vi "BRig_FPGA_stateSelection_laserEvent.vi"(0 "I_LR_reward":bool, 1 "I_LR_reward_laser":bool, 3 "I_LR_wrong":bool, 4 "I_LR_wrong_laser":bool, 6 "I_selectWrong":bool, 7 "laser_reward_nTotal":u32=100, 8 "I_selectReward":bool, 9 "laser_reward_nDelay":u32, 10 "counter":u32, 11 "laser_wrong_nTotal":u32=100, 13 "laser_wrong_nDelay":u32) -> (12 "output_counter":u32, 15 "output_I_laserEvent":bool, 17 "output_I_laserOn":bool)   [LabVIEW 2014]
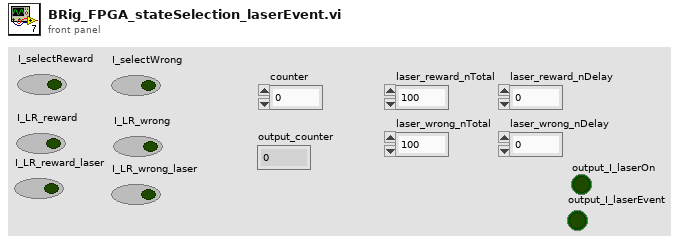
[diagram p1: front panel]
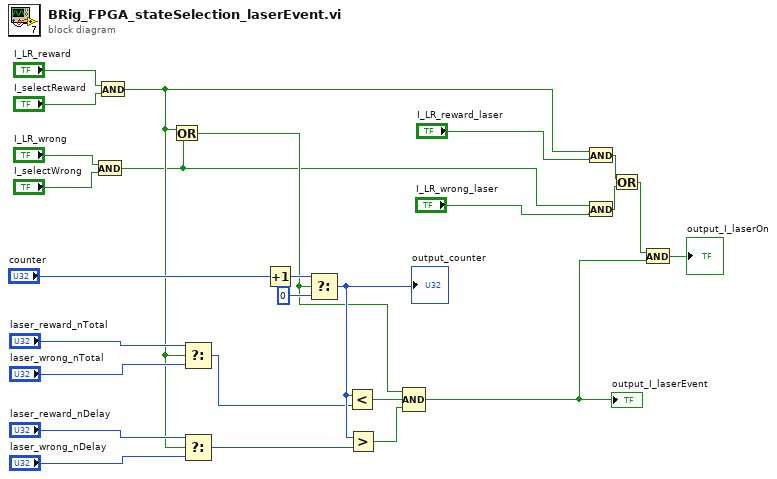
[diagram p0: block diagram]
diagram:
  n1 = And(x="I_LR_wrong", y="I_selectWrong") -> (x .and. y?=w6:bool)
  n2 = And(x="I_LR_reward", y="I_selectReward") -> (x .and. y?=w9:bool)
  n3 = Or(x=w9, y=w6) -> (x .or. y?=w10:bool)
  n4 = Select(t="laser_reward_nTotal", s=w9, f="laser_wrong_nTotal") -> (s? t:f=w13:u32)
  n5 = Select(t="laser_reward_nDelay", s=w9, f="laser_wrong_nDelay") -> (s? t:f=w18:u32)
  n6 = Increment(x="counter") -> (x+1=w22:u32)
  n7 = Select(t=w22, s=w10, f=u32 0) -> (s? t:f=w19:u32)
  "output_counter" <- w19
  n8 = Less?(x=w19, y=w13) -> (x < y?=w11:bool)
  n9 = Greater?(x=w19, y=w18) -> (0:w12:bool)
  n10 = Compound Arithmetic op=AND(w10, w11, w12) -> (w3:bool)
  "output_I_laserEvent" <- w3
  n11 = And(x=w9, y="I_LR_reward_laser") -> (x .and. y?=w4:bool)
  n12 = And(x=w6, y="I_LR_wrong_laser") -> (x .and. y?=w5:bool)
  n13 = Or(x=w4, y=w5) -> (x .or. y?=w2:bool)
  n14 = And(x=w2, y=w3) -> (x .and. y?=→"output_I_laserOn":bool)
